vi "sub vi - Read Analog All v6.vi"() -> (2 "Analog loop time":dbl, 3 "array GRAPH":dynamicdata[](array[waveform]), 4 "array LAB01":dbl[](array[numeric]), 6 "array LAB02":dbl[](array[numeric]), 8 "array LAB03":dbl[](array[numeric]), 10 "array LAB04":dbl[](array[numeric]), 14 "array ERROR":errorcluster[](array[cluster]), 15 "array LAB05":dbl[](array[numeric]))   [LabVIEW 2013]
uses:
  <vilib>/addons/Electrical Power/Basic/Measurement/Power (1 Channel).vi
  <vilib>/addons/Electrical Power/Basic/Measurement/RMS (N Channels).vi
  <vilib>/addons/Electrical Power/Basic/NI_EP_Basic.lvlib
panel:
  in  "Tab Control":T1(tab)
  out "LAB01-2 (PF)":dbl
  out "LAB01-1 (PF)":dbl
  out "LAB01-2 (V)":dbl
  out "LAB01-2 (A)":dbl
  out "LAB01-1 (V)":dbl
  out "LAB01-1 (A)":dbl
  out "LAB01-2 (GRAPH)":dynamicdata(graph)
  out "LAB01-1 (GRAPH)":dynamicdata(graph)
  out "LAB02-2 (PF)":dbl
  out "LAB02-1 (PF)":dbl
  out "LAB02-2 (V)":dbl
  out "LAB02-2 (A)":dbl
  out "LAB02-1 (V)":dbl
  out "LAB02-1 (A)":dbl
  out "LAB02-2 (GRAPH)":dynamicdata(graph)
  out "LAB02-1 (GRAPH)":dynamicdata(graph)
  out "LAB03-2 (PF)":dbl
  out "LAB03-1 (PF)":dbl
  out "LAB03-2 (V)":dbl
  out "LAB03-2 (A)":dbl
  out "LAB03-1 (V)":dbl
  out "LAB03-1 (A)":dbl
  out "LAB03-2 (GRAPH)":dynamicdata(graph)
  out "LAB03-1 (GRAPH)":dynamicdata(graph)
  out "LAB04-2 (PF)":dbl
  out "LAB04-1 (PF)":dbl
  out "LAB04-2 (V)":dbl
  out "LAB04-2 (A)":dbl
  out "LAB04-1 (V)":dbl
  out "LAB04-1 (A)":dbl
  out "LAB04-1 (GRAPH)":dynamicdata(graph)
  out "LAB04-2 (GRAPH)":dynamicdata(graph)
  out "LAB05-2 (PF)":dbl
  out "LAB05-1 (PF)":dbl
  out "LAB05-2 (V)":dbl
  out "LAB05-2 (A)":dbl
  out "LAB05-1 (V)":dbl
  out "LAB05-1 (A)":dbl
  out "LAB05-1 (GRAPH)":dynamicdata(graph)
  out "LAB05-2 (GRAPH)":dynamicdata(graph)
  # "-1 (A)"
  # "-1 (V)"
  # "-1 (PF)"
  # "-2 (A)"
  # "-2 (V)"
  # "-2 (PF)"
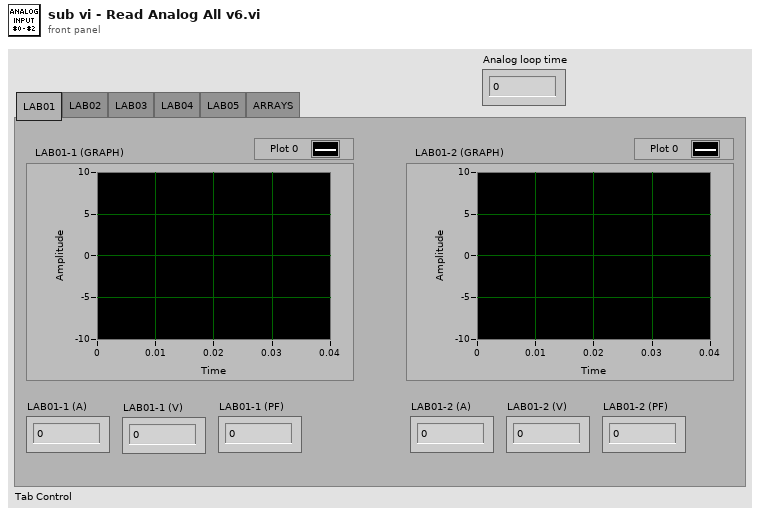
[diagram p1: front panel]
types:
  T1 = enum32{"LAB01", "LAB02", "LAB03", "LAB04", "LAB05", "ARRAYS"}
  T2 = typedef "NI_EP_Basic.lvlib/basic_Power Value.ctl" = cluster{"active power [W]":dbl, "apparent power [VA]":dbl, "reactive power [VAR]":dbl, "power factor":dbl}
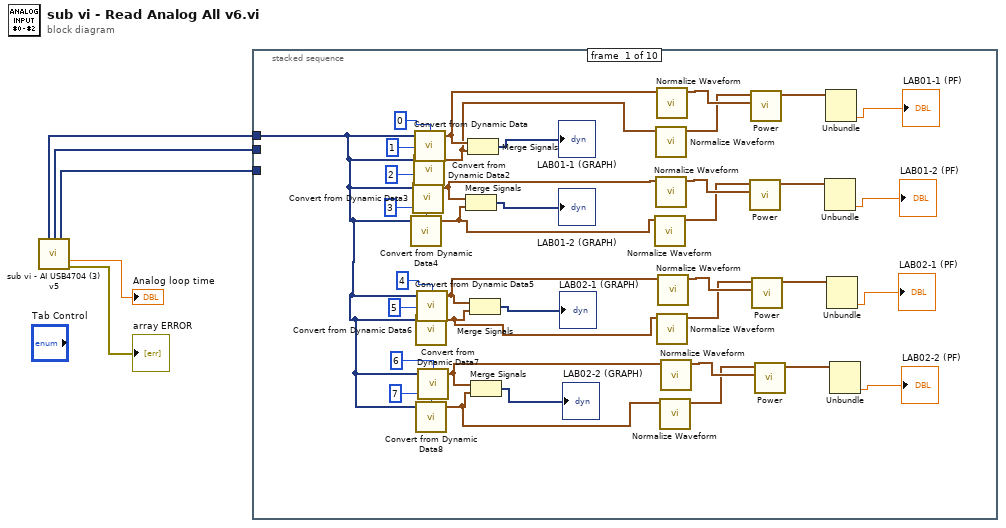
[diagram p0: block diagram]
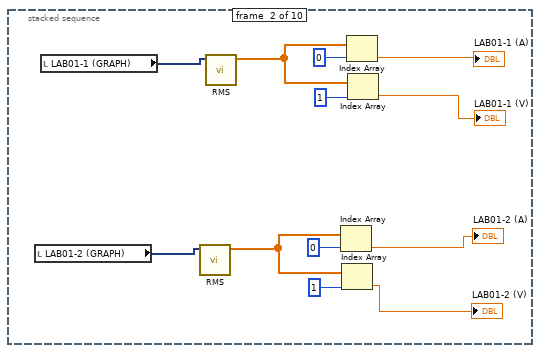
[diagram p2: hidden frame]
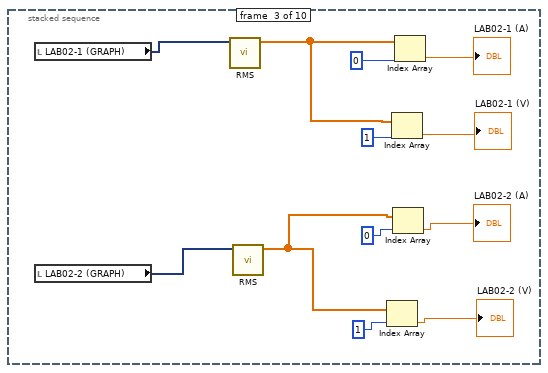
[diagram p3: hidden frame]
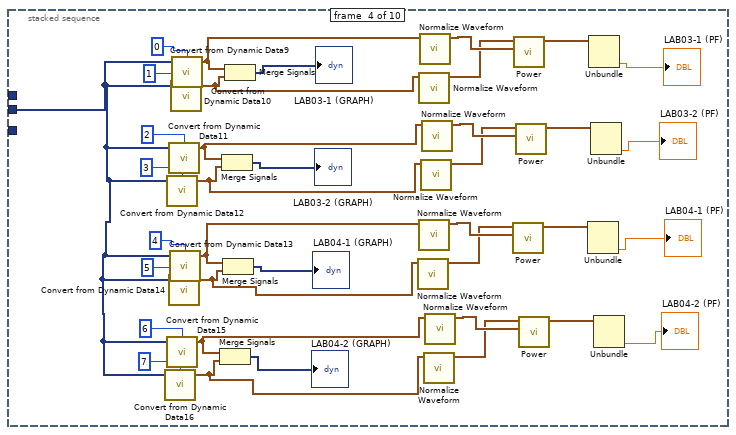
[diagram p4: hidden frame]
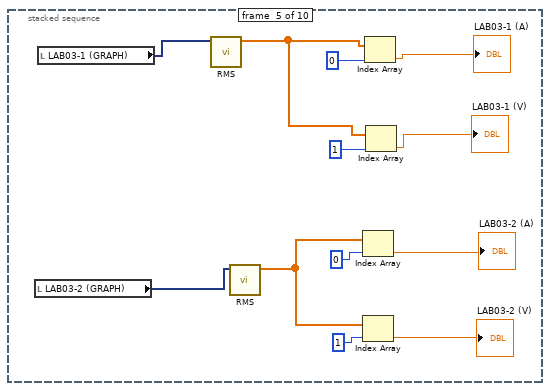
[diagram p5: hidden frame]
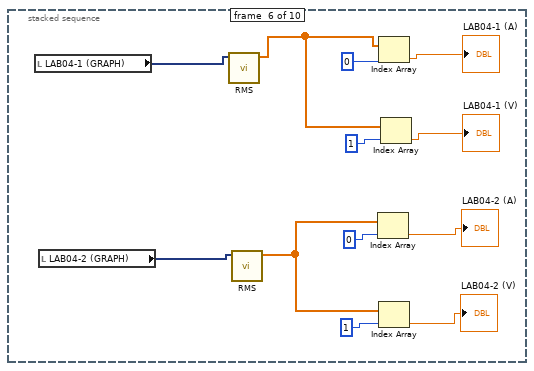
[diagram p6: hidden frame]
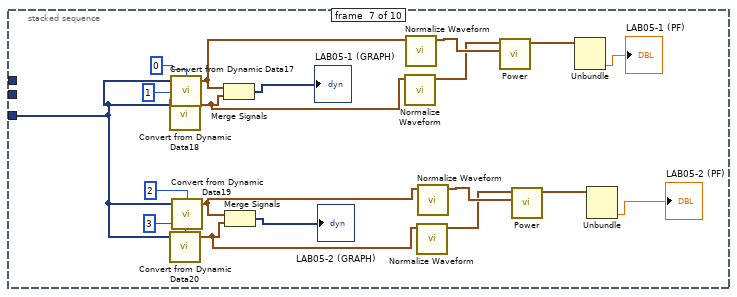
[diagram p7: hidden frame]
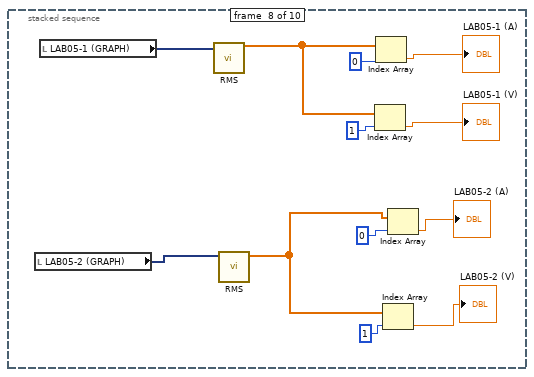
[diagram p8: hidden frame]
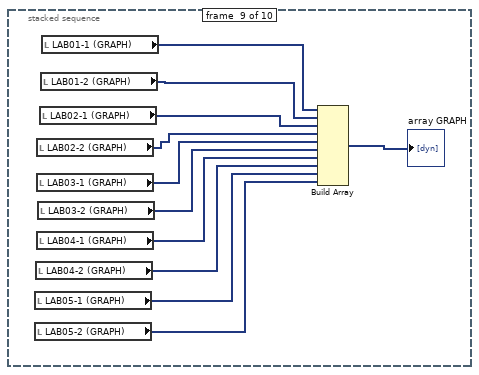
[diagram p9: hidden frame]
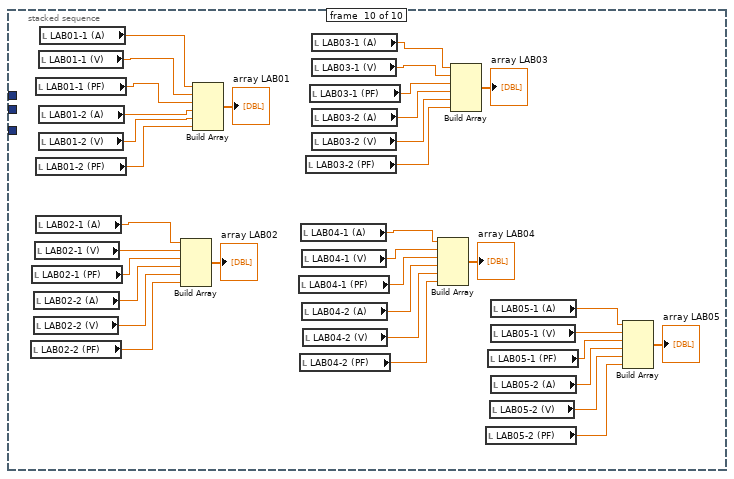
[diagram p10: hidden frame]
diagram:
  n1 = call "sub vi - AI USB4704 (3) v5.vi"() -> ("Graph 1"=w5:dynamicdata, "Graph 2"=w4:dynamicdata, "Graph 3"=w3:dynamicdata, "loop time"=→"Analog loop time":dbl, "error array"=→"array ERROR":errorcluster[])  [unwired: 11 in]
  n2 = stacked-sequence {
    tunnel: w5 -> [w32 _ _ _ _ _ _ _ _ _]
    tunnel: w4 -> [_ _ _ w91 _ _ _ _ _ _]
    tunnel: w3 -> [_ _ _ _ _ _ w140 _ _ _]
    frame #0 {
      n3 = call "Convert from Dynamic Data4"("Dynamic Data Type"=w32, "Channel"=3) -> ("Waveform"=w18:waveform(dbl))  [unwired: 2 in]
      n4 = call "Convert from Dynamic Data3"("Dynamic Data Type"=w32, "Channel"=2) -> ("Waveform"=w19:waveform(dbl))  [unwired: 2 in]
      n5 = call "Convert from Dynamic Data2"("Dynamic Data Type"=w32, "Channel"=1) -> ("Waveform"=w28:waveform(dbl))  [unwired: 2 in]
      n6 = call "Convert from Dynamic Data"("Dynamic Data Type"=w32, "Channel"=0) -> ("Waveform"=w29:waveform(dbl))  [unwired: 2 in]
      n7 = call "Convert from Dynamic Data6"("Dynamic Data Type"=w32, "Channel"=5) -> ("Waveform"=w13:waveform(dbl))  [unwired: 2 in]
      n8 = call "Convert from Dynamic Data8"("Dynamic Data Type"=w32, "Channel"=7) -> ("Waveform"=w7:waveform(dbl))  [unwired: 2 in]
      n9 = call "Convert from Dynamic Data5"("Dynamic Data Type"=w32, "Channel"=4) -> ("Waveform"=w14:waveform(dbl))  [unwired: 2 in]
      n10 = call "Convert from Dynamic Data7"("Dynamic Data Type"=w32, "Channel"=6) -> ("Waveform"=w8:waveform(dbl))  [unwired: 2 in]
      n11 = Merge Signals(w19, w18) -> (→"LAB01-2 (GRAPH)":dynamicdata)
      n12 = Merge Signals(w29, w28) -> (→"LAB01-1 (GRAPH)":dynamicdata)
      n13 = Merge Signals(w14, w13) -> (→"LAB02-1 (GRAPH)":dynamicdata)
      n14 = Merge Signals(w8, w7) -> (→"LAB02-2 (GRAPH)":dynamicdata)
      n15 = call <vilib>:"Normalize Waveform.vi"("waveform in"=w18) -> ("normalized waveform"=w22:waveform(dbl))  [unwired: 7 in, 3 out]
      n16 = call <vilib>:"Normalize Waveform.vi"("waveform in"=w28) -> ("normalized waveform"=w26:waveform(dbl))  [unwired: 7 in, 3 out]
      n17 = call <vilib>:"Normalize Waveform.vi"("waveform in"=w19) -> ("normalized waveform"=w23:waveform(dbl))  [unwired: 7 in, 3 out]
      n18 = call <vilib>:"Normalize Waveform.vi"("waveform in"=w29) -> ("normalized waveform"=w27:waveform(dbl))  [unwired: 7 in, 3 out]
      n19 = call <vilib>:"Normalize Waveform.vi"("waveform in"=w13) -> ("normalized waveform"=w16:waveform(dbl))  [unwired: 7 in, 3 out]
      n20 = call <vilib>:"Normalize Waveform.vi"("waveform in"=w14) -> ("normalized waveform"=w17:waveform(dbl))  [unwired: 7 in, 3 out]
      n21 = call <vilib>:"Normalize Waveform.vi"("waveform in"=w7) -> ("normalized waveform"=w10:waveform(dbl))  [unwired: 7 in, 3 out]
      n22 = call <vilib>:"Normalize Waveform.vi"("waveform in"=w8) -> ("normalized waveform"=w11:waveform(dbl))  [unwired: 7 in, 3 out]
      n23 = call-poly <vilib>:"Power.vi"("current waveform"=w23, "voltage waveform"=w22) -> ("power value"=w21:T2)  [unwired: 8 in, 1 out]
      n24 = call-poly <vilib>:"Power.vi"("current waveform"=w27, "voltage waveform"=w26) -> ("power value"=w25:T2)  [unwired: 8 in, 1 out]
      n25 = call-poly <vilib>:"Power.vi"("current waveform"=w17, "voltage waveform"=w16) -> ("power value"=w15:T2)  [unwired: 8 in, 1 out]
      n26 = call-poly <vilib>:"Power.vi"("current waveform"=w11, "voltage waveform"=w10) -> ("power value"=w9:T2)  [unwired: 8 in, 1 out]
      n27 = Unbundle(w21) -> ("power factor"=→"LAB01-2 (PF)":dbl)  [unwired: 3 out]
      n28 = Unbundle(w25) -> ("power factor"=→"LAB01-1 (PF)":dbl)  [unwired: 3 out]
      n29 = Unbundle(w15) -> ("power factor"=→"LAB02-1 (PF)":dbl)  [unwired: 3 out]
      n30 = Unbundle(w9) -> ("power factor"=→"LAB02-2 (PF)":dbl)  [unwired: 3 out]
    }
    frame #1 {
      n31 = local read "LAB01-2 (GRAPH)"() -> (w51:dynamicdata)
      n32 = local read "LAB01-1 (GRAPH)"() -> (w45:dynamicdata)
      n33 = call-poly <vilib>:"RMS.vi"("waveforms"=w51) -> ("RMS values"=w50:dbl[])  [unwired: 9 in, 1 out]
      n34 = call-poly <vilib>:"RMS.vi"("waveforms"=w45) -> ("RMS values"=w54:dbl[])  [unwired: 9 in, 1 out]
      n35 = Index Array(array=w50, index=0) -> (element=→"LAB01-2 (A)":dbl)
      n36 = Index Array(array=w50, index=1) -> (element=→"LAB01-2 (V)":dbl)
      n37 = Index Array(array=w54, index=0) -> (element=→"LAB01-1 (A)":dbl)
      n38 = Index Array(array=w54, index=1) -> (element=→"LAB01-1 (V)":dbl)
    }
    frame #2 {
      n39 = local read "LAB02-1 (GRAPH)"() -> (w62:dynamicdata)
      n40 = local read "LAB02-2 (GRAPH)"() -> (w58:dynamicdata)
      n41 = call-poly <vilib>:"RMS.vi"("waveforms"=w62) -> ("RMS values"=w61:dbl[])  [unwired: 9 in, 1 out]
      n42 = call-poly <vilib>:"RMS.vi"("waveforms"=w58) -> ("RMS values"=w57:dbl[])  [unwired: 9 in, 1 out]
      n43 = Index Array(array=w57, index=1) -> (element=→"LAB02-2 (V)":dbl)
      n44 = Index Array(array=w61, index=1) -> (element=→"LAB02-1 (V)":dbl)
      n45 = Index Array(array=w57, index=0) -> (element=→"LAB02-2 (A)":dbl)
      n46 = Index Array(array=w61, index=0) -> (element=→"LAB02-1 (A)":dbl)
    }
    frame #3 {
      n47 = call "Convert from Dynamic Data16"("Dynamic Data Type"=w91, "Channel"=7) -> ("Waveform"=w68:waveform(dbl))  [unwired: 2 in]
      n48 = call "Convert from Dynamic Data12"("Dynamic Data Type"=w91, "Channel"=3) -> ("Waveform"=w80:waveform(dbl))  [unwired: 2 in]
      n49 = call "Convert from Dynamic Data15"("Dynamic Data Type"=w91, "Channel"=6) -> ("Waveform"=w69:waveform(dbl))  [unwired: 2 in]
      n50 = call "Convert from Dynamic Data11"("Dynamic Data Type"=w91, "Channel"=2) -> ("Waveform"=w81:waveform(dbl))  [unwired: 2 in]
      n51 = call "Convert from Dynamic Data14"("Dynamic Data Type"=w91, "Channel"=5) -> ("Waveform"=w74:waveform(dbl))  [unwired: 2 in]
      n52 = call "Convert from Dynamic Data13"("Dynamic Data Type"=w91, "Channel"=4) -> ("Waveform"=w75:waveform(dbl))  [unwired: 2 in]
      n53 = call "Convert from Dynamic Data10"("Dynamic Data Type"=w91, "Channel"=1) -> ("Waveform"=w86:waveform(dbl))  [unwired: 2 in]
      n54 = call "Convert from Dynamic Data9"("Dynamic Data Type"=w91, "Channel"=0) -> ("Waveform"=w87:waveform(dbl))  [unwired: 2 in]
      n55 = Merge Signals(w69, w68) -> (→"LAB04-2 (GRAPH)":dynamicdata)
      n56 = Merge Signals(w81, w80) -> (→"LAB03-2 (GRAPH)":dynamicdata)
      n57 = Merge Signals(w75, w74) -> (→"LAB04-1 (GRAPH)":dynamicdata)
      n58 = Merge Signals(w87, w86) -> (→"LAB03-1 (GRAPH)":dynamicdata)
      n59 = call <vilib>:"Normalize Waveform.vi"("waveform in"=w74) -> ("normalized waveform"=w77:waveform(dbl))  [unwired: 7 in, 3 out]
      n60 = call <vilib>:"Normalize Waveform.vi"("waveform in"=w86) -> ("normalized waveform"=w89:waveform(dbl))  [unwired: 7 in, 3 out]
      n61 = call <vilib>:"Normalize Waveform.vi"("waveform in"=w75) -> ("normalized waveform"=w78:waveform(dbl))  [unwired: 7 in, 3 out]
      n62 = call <vilib>:"Normalize Waveform.vi"("waveform in"=w87) -> ("normalized waveform"=w90:waveform(dbl))  [unwired: 7 in, 3 out]
      n63 = call <vilib>:"Normalize Waveform.vi"("waveform in"=w80) -> ("normalized waveform"=w83:waveform(dbl))  [unwired: 7 in, 3 out]
      n64 = call <vilib>:"Normalize Waveform.vi"("waveform in"=w81) -> ("normalized waveform"=w84:waveform(dbl))  [unwired: 7 in, 3 out]
      n65 = call <vilib>:"Normalize Waveform.vi"("waveform in"=w68) -> ("normalized waveform"=w71:waveform(dbl))  [unwired: 7 in, 3 out]
      n66 = call <vilib>:"Normalize Waveform.vi"("waveform in"=w69) -> ("normalized waveform"=w72:waveform(dbl))  [unwired: 7 in, 3 out]
      n67 = call-poly <vilib>:"Power.vi"("current waveform"=w78, "voltage waveform"=w77) -> ("power value"=w76:T2)  [unwired: 8 in, 1 out]
      n68 = call-poly <vilib>:"Power.vi"("current waveform"=w90, "voltage waveform"=w89) -> ("power value"=w88:T2)  [unwired: 8 in, 1 out]
      n69 = call-poly <vilib>:"Power.vi"("current waveform"=w84, "voltage waveform"=w83) -> ("power value"=w82:T2)  [unwired: 8 in, 1 out]
      n70 = call-poly <vilib>:"Power.vi"("current waveform"=w72, "voltage waveform"=w71) -> ("power value"=w70:T2)  [unwired: 8 in, 1 out]
      n71 = Unbundle(w76) -> ("power factor"=→"LAB04-1 (PF)":dbl)  [unwired: 3 out]
      n72 = Unbundle(w88) -> ("power factor"=→"LAB03-1 (PF)":dbl)  [unwired: 3 out]
      n73 = Unbundle(w82) -> ("power factor"=→"LAB03-2 (PF)":dbl)  [unwired: 3 out]
      n74 = Unbundle(w70) -> ("power factor"=→"LAB04-2 (PF)":dbl)  [unwired: 3 out]
    }
    frame #4 {
      n75 = local read "LAB03-2 (GRAPH)"() -> (w110:dynamicdata)
      n76 = local read "LAB03-1 (GRAPH)"() -> (w111:dynamicdata)
      n77 = call-poly <vilib>:"RMS.vi"("waveforms"=w111) -> ("RMS values"=w109:dbl[])  [unwired: 9 in, 1 out]
      n78 = call-poly <vilib>:"RMS.vi"("waveforms"=w110) -> ("RMS values"=w106:dbl[])  [unwired: 9 in, 1 out]
      n79 = Index Array(array=w106, index=0) -> (element=→"LAB03-2 (A)":dbl)
      n80 = Index Array(array=w106, index=1) -> (element=→"LAB03-2 (V)":dbl)
      n81 = Index Array(array=w109, index=0) -> (element=→"LAB03-1 (A)":dbl)
      n82 = Index Array(array=w109, index=1) -> (element=→"LAB03-1 (V)":dbl)
    }
    frame #5 {
      n83 = local read "LAB04-1 (GRAPH)"() -> (w123:dynamicdata)
      n84 = local read "LAB04-2 (GRAPH)"() -> (w119:dynamicdata)
      n85 = call-poly <vilib>:"RMS.vi"("waveforms"=w123) -> ("RMS values"=w122:dbl[])  [unwired: 9 in, 1 out]
      n86 = call-poly <vilib>:"RMS.vi"("waveforms"=w119) -> ("RMS values"=w118:dbl[])  [unwired: 9 in, 1 out]
      n87 = Index Array(array=w118, index=0) -> (element=→"LAB04-2 (A)":dbl)
      n88 = Index Array(array=w122, index=0) -> (element=→"LAB04-1 (A)":dbl)
      n89 = Index Array(array=w118, index=1) -> (element=→"LAB04-2 (V)":dbl)
      n90 = Index Array(array=w122, index=1) -> (element=→"LAB04-1 (V)":dbl)
    }
    frame #6 {
      n91 = call "Convert from Dynamic Data18"("Dynamic Data Type"=w140, "Channel"=1) -> ("Waveform"=w135:waveform(dbl))  [unwired: 2 in]
      n92 = call "Convert from Dynamic Data20"("Dynamic Data Type"=w140, "Channel"=3) -> ("Waveform"=w129:waveform(dbl))  [unwired: 2 in]
      n93 = call "Convert from Dynamic Data17"("Dynamic Data Type"=w140, "Channel"=0) -> ("Waveform"=w136:waveform(dbl))  [unwired: 2 in]
      n94 = call "Convert from Dynamic Data19"("Dynamic Data Type"=w140, "Channel"=2) -> ("Waveform"=w130:waveform(dbl))  [unwired: 2 in]
      n95 = Merge Signals(w136, w135) -> (→"LAB05-1 (GRAPH)":dynamicdata)
      n96 = Merge Signals(w130, w129) -> (→"LAB05-2 (GRAPH)":dynamicdata)
      n97 = call <vilib>:"Normalize Waveform.vi"("waveform in"=w135) -> ("normalized waveform"=w138:waveform(dbl))  [unwired: 7 in, 3 out]
      n98 = call <vilib>:"Normalize Waveform.vi"("waveform in"=w136) -> ("normalized waveform"=w139:waveform(dbl))  [unwired: 7 in, 3 out]
      n99 = call <vilib>:"Normalize Waveform.vi"("waveform in"=w129) -> ("normalized waveform"=w132:waveform(dbl))  [unwired: 7 in, 3 out]
      n100 = call <vilib>:"Normalize Waveform.vi"("waveform in"=w130) -> ("normalized waveform"=w133:waveform(dbl))  [unwired: 7 in, 3 out]
      n101 = call-poly <vilib>:"Power.vi"("current waveform"=w139, "voltage waveform"=w138) -> ("power value"=w137:T2)  [unwired: 8 in, 1 out]
      n102 = call-poly <vilib>:"Power.vi"("current waveform"=w133, "voltage waveform"=w132) -> ("power value"=w131:T2)  [unwired: 8 in, 1 out]
      n103 = Unbundle(w137) -> ("power factor"=→"LAB05-1 (PF)":dbl)  [unwired: 3 out]
      n104 = Unbundle(w131) -> ("power factor"=→"LAB05-2 (PF)":dbl)  [unwired: 3 out]
    }
    frame #7 {
      n105 = local read "LAB05-2 (GRAPH)"() -> (w153:dynamicdata)
      n106 = local read "LAB05-1 (GRAPH)"() -> (w154:dynamicdata)
      n107 = call-poly <vilib>:"RMS.vi"("waveforms"=w154) -> ("RMS values"=w152:dbl[])  [unwired: 9 in, 1 out]
      n108 = call-poly <vilib>:"RMS.vi"("waveforms"=w153) -> ("RMS values"=w151:dbl[])  [unwired: 9 in, 1 out]
      n109 = Index Array(array=w152, index=1) -> (element=→"LAB05-1 (V)":dbl)
      n110 = Index Array(array=w152, index=0) -> (element=→"LAB05-1 (A)":dbl)
      n111 = Index Array(array=w151, index=1) -> (element=→"LAB05-2 (V)":dbl)
      n112 = Index Array(array=w151, index=0) -> (element=→"LAB05-2 (A)":dbl)
    }
    frame #8 {
      n113 = local read "LAB05-1 (GRAPH)"() -> (w161:dynamicdata)
      n114 = local read "LAB05-2 (GRAPH)"() -> (w160:dynamicdata)
      n115 = local read "LAB04-2 (GRAPH)"() -> (w162:dynamicdata)
      n116 = local read "LAB02-2 (GRAPH)"() -> (w166:dynamicdata)
      n117 = local read "LAB03-1 (GRAPH)"() -> (w165:dynamicdata)
      n118 = local read "LAB04-1 (GRAPH)"() -> (w163:dynamicdata)
      n119 = local read "LAB03-2 (GRAPH)"() -> (w164:dynamicdata)
      n120 = local read "LAB02-1 (GRAPH)"() -> (w167:dynamicdata)
      n121 = local read "LAB01-2 (GRAPH)"() -> (w168:dynamicdata)
      n122 = local read "LAB01-1 (GRAPH)"() -> (w169:dynamicdata)
      n123 = Build Array(w169, w168, w167, w166, w165, w164, w163, w162, w161, w160) -> (→"array GRAPH":dynamicdata[])
    }
    frame #9 {
      n124 = local read "LAB02-2 (PF)"() -> (w192:dbl)
      n125 = local read "LAB02-1 (PF)"() -> (w195:dbl)
      n126 = local read "LAB02-2 (A)"() -> (w194:dbl)
      n127 = local read "LAB02-2 (V)"() -> (w193:dbl)
      n128 = local read "LAB02-1 (V)"() -> (w196:dbl)
      n129 = local read "LAB01-1 (PF)"() -> (w202:dbl)
      n130 = local read "LAB01-2 (PF)"() -> (w199:dbl)
      n131 = local read "LAB02-1 (A)"() -> (w197:dbl)
      n132 = local read "LAB01-1 (V)"() -> (w203:dbl)
      n133 = local read "LAB01-2 (A)"() -> (w201:dbl)
      n134 = local read "LAB01-2 (V)"() -> (w200:dbl)
      n135 = local read "LAB01-1 (A)"() -> (w204:dbl)
      n136 = Build Array(w197, w196, w195, w194, w193, w192) -> (→"array LAB02":dbl[])
      n137 = Build Array(w204, w203, w202, w201, w200, w199) -> (→"array LAB01":dbl[])
      n138 = local read "LAB04-1 (PF)"() -> (w181:dbl)
      n139 = local read "LAB04-2 (PF)"() -> (w178:dbl)
      n140 = local read "LAB04-1 (A)"() -> (w183:dbl)
      n141 = local read "LAB04-1 (V)"() -> (w182:dbl)
      n142 = local read "LAB04-2 (A)"() -> (w180:dbl)
      n143 = local read "LAB04-2 (V)"() -> (w179:dbl)
      n144 = local read "LAB03-2 (PF)"() -> (w185:dbl)
      n145 = local read "LAB03-1 (PF)"() -> (w188:dbl)
      n146 = local read "LAB03-1 (A)"() -> (w190:dbl)
      n147 = local read "LAB03-1 (V)"() -> (w189:dbl)
      n148 = local read "LAB03-2 (A)"() -> (w187:dbl)
      n149 = local read "LAB03-2 (V)"() -> (w186:dbl)
      n150 = Build Array(w183, w182, w181, w180, w179, w178) -> (→"array LAB04":dbl[])
      n151 = Build Array(w190, w189, w188, w187, w186, w185) -> (→"array LAB03":dbl[])
      n152 = local read "LAB05-2 (PF)"() -> (w171:dbl)
      n153 = local read "LAB05-1 (PF)"() -> (w174:dbl)
      n154 = local read "LAB05-2 (V)"() -> (w172:dbl)
      n155 = local read "LAB05-1 (A)"() -> (w176:dbl)
      n156 = local read "LAB05-1 (V)"() -> (w175:dbl)
      n157 = local read "LAB05-2 (A)"() -> (w173:dbl)
      n158 = Build Array(w176, w175, w174, w173, w172, w171) -> (→"array LAB05":dbl[])
    }
  }
